vi "Camera - Sequence Program.vi"() -> ()   [LabVIEW 2014]
uses:
  Camera Settings.ctl
  Camera Refnums.ctl
  Camera Functions.ctl
panel:
  in  "Video":bool
  out "Image":T1(plugin-control)
  in  "Settings":T2={"Pixel clock"=20, "Frame rate"=30.0, "Exposure time"=33.21525, "Master Gain"=0, "Red Gain"=0, "Green Gain"=0, "Blue Gain"=0, "Auto Gain"=FALSE, "White-balance"=FALSE, "Color Correction"=FALSE} {"Blue Gain" min=0 max=100 step=1 scale=0.0..100.0; "Green Gain" min=0 max=100 step=1 scale=0.0..100.0; "Red Gain" min=0 max=100 step=1 scale=0.0..100.0; "Master Gain" min=0 max=100 step=1 scale=0.0..100.0; "Exposure time" min=0.12195 max=191.09565 step=0.12195 scale=0.12195..191.09565 scale format="%#.3g"; "Frame rate" min=2.744797322450212 max=5.222982166127394 step=0.00012195 scale=5.222982166127394..5.745280382740133 scale format="%^#_3g"; "Pixel clock" min=5 max=43 step=1 scale=5.0..43.0}
  out "Error Out":errorcluster
  in  "Quit":bool
  # "LICENSED MATERIALS – PROPERTY OF IBM\nCopyright IBM Corp. 2016,\nALL RIGHTS RESERVED"
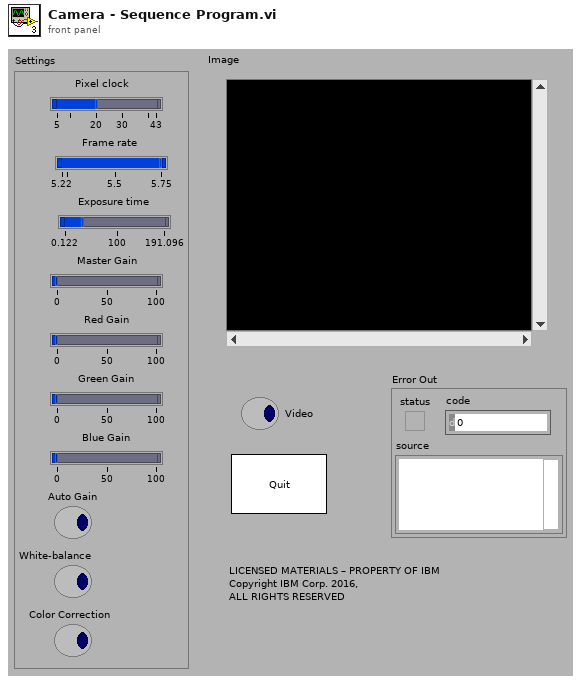
[diagram p1: front panel]
types:
  T1 = typedef "IMAQ Image.ctl" = refnum<image>
  T2 = typedef "Camera Settings.ctl" = cluster{"Pixel clock":i32, "Frame rate":dbl, "Exposure time":dbl, "Master Gain":i32, "Red Gain":i32, "Green Gain":i32, "Blue Gain":i32, "Auto Gain":bool, "White-balance":bool, "Color Correction":bool}
  T3 = typedef "Camera Functions.ctl" = enum16{"Connect", "Start Live", "Acquire", "Update Settings", "Update Settings2", "Stop Live", "Disconnect", "Update Refnums"}
  T4 = typedef "Camera Refnums.ctl" = cluster{"Pixel Clock":refnum<vi>, "Frame Rate":refnum<vi>, "Exposure Time":refnum<vi>, "Master Gain":refnum<vi>, "Red Gain":refnum<vi>, "Green Gain":refnum<vi>, "Blue Gain":refnum<vi>, "Auto Gain":refnum<vi>, "Auto White-balance":refnum<vi>, "Color Correction":refnum<vi>, "Image":refnum<vi>, "Video Button":refnum<vi>, "Instrument Status":refnum<vi>}
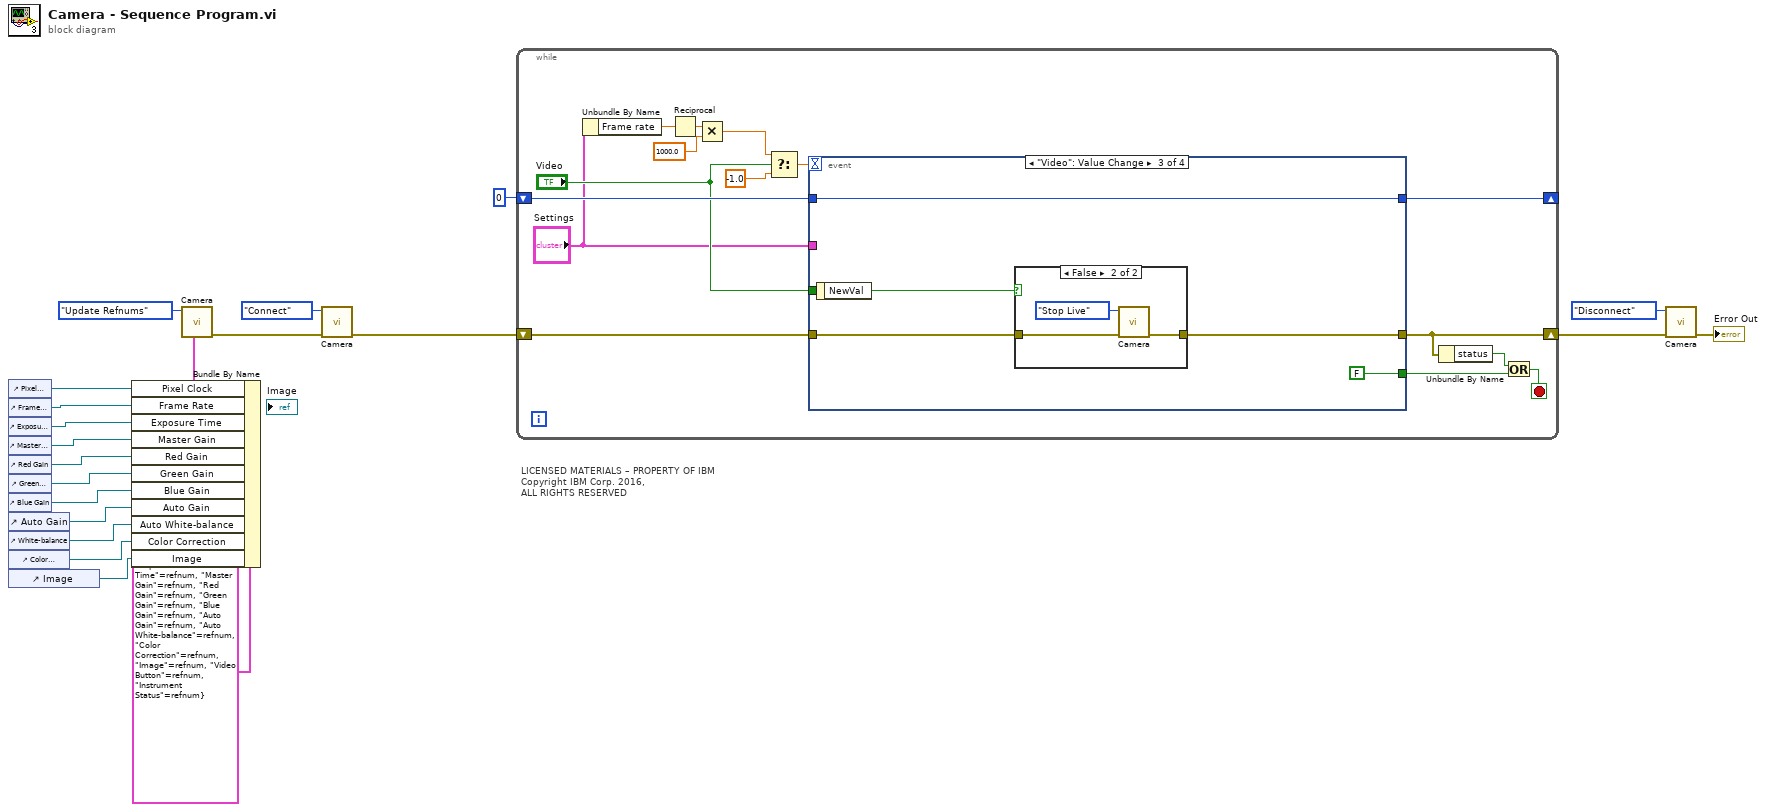
[diagram p0: block diagram]
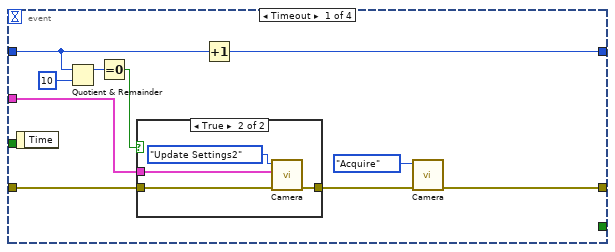
[diagram p2: hidden frame]
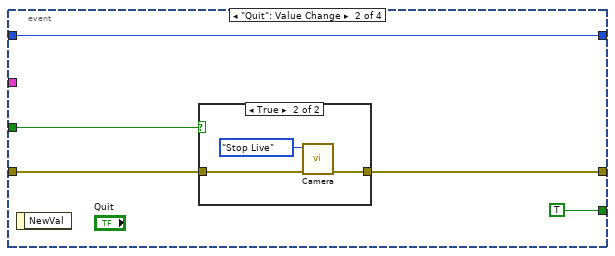
[diagram p4: hidden frame]
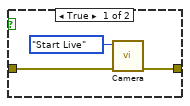
[diagram p6: hidden frame]
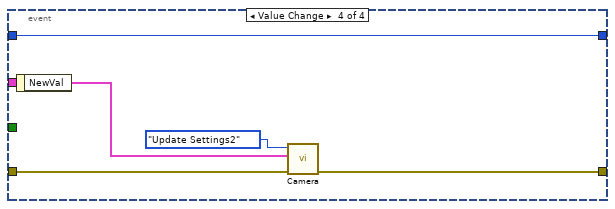
[diagram p7: hidden frame]
diagram:
  # "LICENSED MATERIALS – PROPERTY OF IBM\nCopyright IBM Corp. 2016,\nALL RIGHTS RESERVED"
  n1 = control-ref of="Pixel clock"() -> (w19:refnum<vi>)
  n2 = control-ref of="Frame rate"() -> (w18:refnum<vi>)
  n3 = control-ref of="Exposure time"() -> (w17:refnum<vi>)
  n4 = control-ref of="Master Gain"() -> (w16:refnum<vi>)
  n5 = control-ref of="Red Gain"() -> (w15:refnum<vi>)
  n6 = control-ref of="Green Gain"() -> (w14:refnum<vi>)
  n7 = control-ref of="Blue Gain"() -> (w13:refnum<vi>)
  n8 = control-ref of="Auto Gain"() -> (w12:refnum<vi>)
  n9 = control-ref of="White-balance"() -> (w11:refnum<vi>)
  n10 = control-ref of="Color Correction"() -> (w10:refnum<vi>)
  n11 = control-ref of="Image"() -> (w9:refnum<vi>)
  n12 = Bundle By Name(cluster=T4 {"Pixel Clock"=refnum, "Frame Rate"=refnum, "Exposure Time"=refnum, "Master Gain"=refnum, "Red Gain"=refnum, "Green Gain"=refnum, "Blue Gain"=refnum, "Auto Gain"=refnum, "Auto White-balance"=refnum, "Color Correction"=refnum, "Image"=refnum, "Video Button"=refnum, "Instrument Status"=refnum} ("Refnums"), "Pixel Clock"=w19, "Frame Rate"=w18, "Exposure Time"=w17, "Master Gain"=w16, "Red Gain"=w15, "Green Gain"=w14, "Blue Gain"=w13, "Auto Gain"=w12, "Auto White-balance"=w11, "Color Correction"=w10, "Image"=w9) -> (w20:T4)
  n13 = call "Camera.vi"("Refnums"=w20, "Function"=Camera_Functions."Update Refnums") -> ("Error Out"=w1:errorcluster)  [unwired: 7 in, 2 out]
  n14 = call "Camera.vi"("Error In"=w1, "Function"=Camera_Functions."Connect") -> ("Error Out"=w2:errorcluster)  [unwired: 7 in, 2 out]
  n15 = while {
    shift-right: [w33] -> w3
    shift-left: w2 -> [w34]
    shift-right: [w27] -> _
    shift-left: 0 -> [w28]
    stop <- w36 stop-if-true
    n16 = Unbundle By Name("Settings") -> ("Frame rate"=w32:dbl)
    n17 = Reciprocal(x=w32) -> (1/x=w31:dbl)
    n18 = Multiply(x=w31, y=1000.0) -> (x*y=w26:dbl)
    n19 = Select(t=w26, s="Video", f=-1.0) -> (s? t:f=w24:dbl)
    n20 = event shown="[2] \"Video\": Value Change" {
      selector: _ -> [_ _ _ _]
      dyn-events: _ -> [_ _ _ _]
      timeout: w24 -> [_ _ _ _]
      tunnel: w34 -> [w41 w54 w63 w76]
      tunnel: [w39 w53 w62 w74] -> w33
      tunnel: [_ TRUE FALSE _] -> w29
      tunnel: w28 -> [w44 w55 w64 w75]
      tunnel: [w46 w55 w64 w75] -> w27
      tunnel: "Settings" -> [w37 _ _ _]
      tunnel: "Video" -> [_ w52 _ _]
      event Timeout {
        n21 = event-data() -> ()  [unwired: 2 out]
        n22 = Quotient & Remainder(x=w44, y=10) -> (x-y*floor(x/y)=w42:i32)  [unwired: 1 out]
        n23 = Equal To 0?(x=w42) -> (x = 0?=w45:bool)
        n24 = case shown="True" w45 {
          tunnel: w41 -> [w47 w51]
          tunnel: [w47 w50] -> w40
          tunnel: w37 -> [_ w48]
          frame False {
          }
          frame True {
            n25 = call "Camera.vi"("Error In"=w51, "Settings"=w48, "Function"=Camera_Functions."Update Settings2") -> ("Error Out"=w50:errorcluster)  [unwired: 6 in, 2 out]
          }
        }
        n26 = Increment(x=w44) -> (x+1=w46:i32)
        n27 = call "Camera.vi"("Error In"=w40, "Function"=Camera_Functions."Acquire") -> ("Error Out"=w39:errorcluster)  [unwired: 7 in, 2 out]
      }
      event "Quit": Value Change {
        n28 = event-data() -> ()  [unwired: 2 out]
        n29 = case shown="True" w52 {
          tunnel: w54 -> [w57 w59]
          tunnel: [w57 w58] -> w53
          frame False {
          }
          frame True {
            n30 = call "Camera.vi"("Error In"=w59, "Function"=Camera_Functions."Stop Live") -> ("Error Out"=w58:errorcluster)  [unwired: 7 in, 2 out]
          }
        }
      }
      event "Video": Value Change {
        n31 = event-data() -> ("NewVal"=w61:bool)  [unwired: 1 out]
        n32 = case shown="False" w61 {
          tunnel: w63 -> [w67 w70]
          tunnel: [w66 w69] -> w62
          frame True {
            n33 = call "Camera.vi"("Error In"=w67, "Function"=Camera_Functions."Start Live") -> ("Error Out"=w66:errorcluster)  [unwired: 7 in, 2 out]
          }
          frame False {
            n34 = call "Camera.vi"("Error In"=w70, "Function"=Camera_Functions."Stop Live") -> ("Error Out"=w69:errorcluster)  [unwired: 7 in, 2 out]
          }
        }
      }
      event Value Change {
        n35 = event-data() -> ("NewVal"=w72:T2)  [unwired: 1 out]
        n36 = call "Camera.vi"("Error In"=w76, "Settings"=w72, "Function"=Camera_Functions."Update Settings2") -> ("Error Out"=w74:errorcluster)  [unwired: 6 in, 2 out]
      }
    }
    n37 = Unbundle By Name(w33) -> ("status"=w35:bool)
    n38 = Or(x=w35, y=w29) -> (x .or. y?=w36:bool)
  }
  n39 = call "Camera.vi"("Error In"=w3, "Function"=Camera_Functions."Disconnect") -> ("Error Out"=→"Error Out":errorcluster)  [unwired: 7 in, 2 out]
